vi "Test VI Type Specifier.vi"(4 "timeout (s) (2000)":i32=2000, 6 "Verbose (F)":bool, 8 "error in":errorcluster, 10 "Interactive (F)":bool, 11 "Report Path":path) -> (0 "error out":errorcluster, 3 "Report Path":path)   [LabVIEW 2020, in "CICD.lvlib"]
doc: "N.B. This VI is non-functional and serves only as a type-specifier for Unit, Integration, and End-to-End tests in the source code."
uses:
  CICD.lvlib
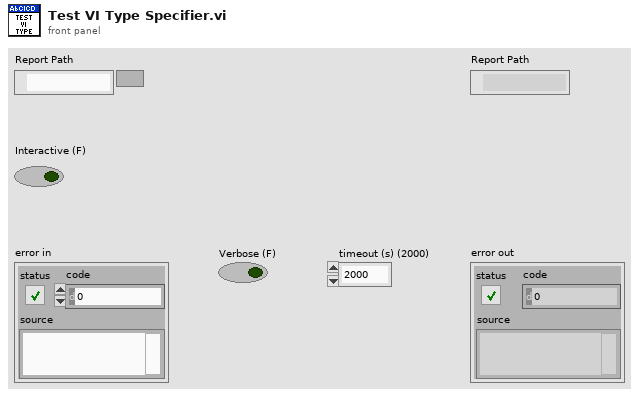
[diagram p1: front panel]
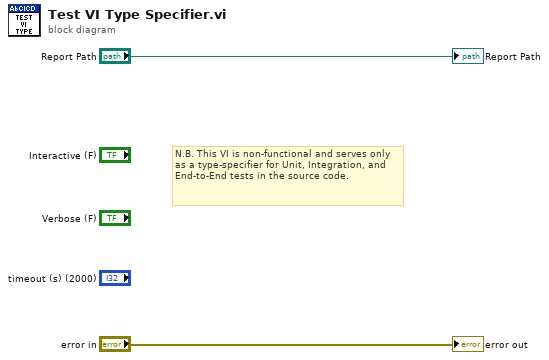
[diagram p0: block diagram]
diagram:
  # "N.B. This VI is non-functional and serves only as a type-specifier for Unit, Integration, and End-to-End tests in the source code."
  "error out" <- "error in"
  "Report Path" <- "Report Path"
